vi "波形发生器子程序.vi"() -> ()   [LabVIEW 2017]
panel:
  out "波形图":waveform(dbl)(graph)
  in  "波形选择":enum16{"公式波", "三角波", "方波", "正弦波"}(ring)
  in  "噪声选择":enum16{"高斯白噪声", "均匀白噪声", "无"}(ring)
  in  "停止":bool
  in  "frequency":dbl=10.0 caption="频率" format="%0.2p"
  in  "amplitude":dbl=1.0 caption="幅值" format="%0.2p"
  in  "phase":dbl caption="相位" format="%.2p"
  in  "square wave duty cycle (%)":dbl=50.0 caption="方波占空比(%)" format="%0.2f"
  in  "信噪比":dbl
  in  "formula":string="sin(w*t)*sin(2*pi(1)*t)" caption="公式"
  in  "sampling info":cluster{"Fs":dbl, "#s":dbl}={"Fs"=1000.0, "#s"=1000.0} caption="采样信息" {"Fs" format="%.2p"}
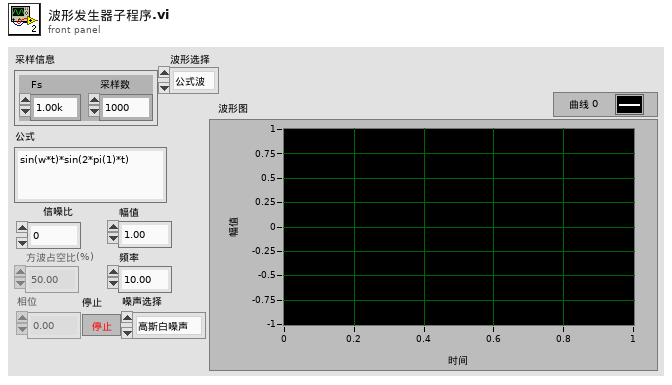
[diagram p1: front panel]
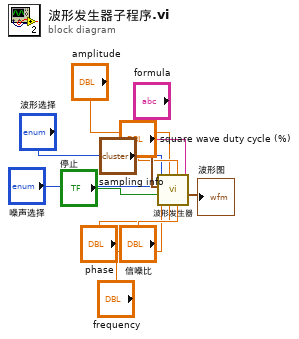
[diagram p0: block diagram]
diagram:
  n1 = call "波形发生器.vi"("sampling info"="sampling info", "formula"="formula", "信噪比"="信噪比", "square wave duty cycle (%)"="square wave duty cycle (%)", "phase"="phase", "amplitude"="amplitude", "frequency"="frequency", "停止"="停止", "噪声选择"="噪声选择", "波形选择"="波形选择") -> ("波形图"=→"波形图":waveform(dbl))  [unwired: 1 in]
